vi "CF_TC to PGSQL.vi"(8 "error in (no error)":errorcluster, 9 "calibration string":string, 10 "description string":string, 11 "dbl":dbl[](array[numeric])) -> (0 "error out":errorcluster)   [LabVIEW 2013]
uses:
  postgreSQL-lv/Data.PG/Data.PGSQL.lvclass
panel:
  # "CF TC to PGSQL"
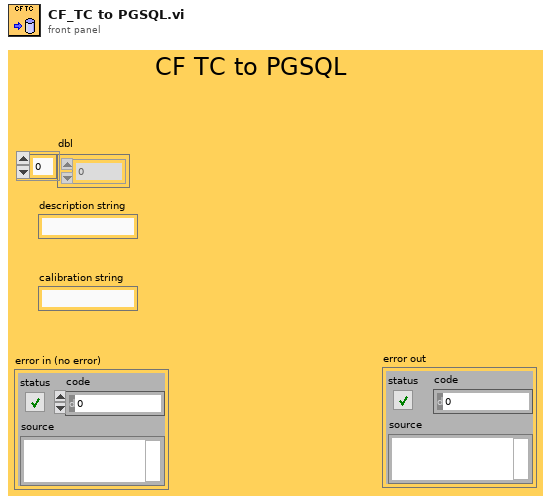
[diagram p1: front panel]
types:
  T1 = cluster{"dbl":dbl[], "description string":string, "calibration string":string}
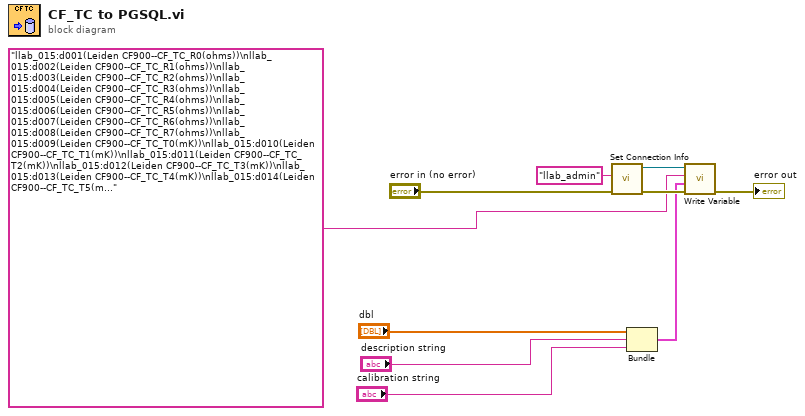
[diagram p0: block diagram]
diagram:
  n1 = call "Set Connection Info.vi"("username"="llab_admin", "error in (no error)"="error in (no error)") -> ("Data.PG out"=w10:refnum<class "Data.PGSQL.lvclass">, "error out"=w9:errorcluster)  [unwired: 7 in]
  n2 = Bundle("dbl"="dbl", "description string"="description string", "calibration string"="calibration string") -> (w7:T1)  [unwired: 1 in]
  n3 = call "Write Variable.vi"("error in (no error)"=w9, "Data"=w7, "variable"="llab_015:d001(Leiden CF900--CF_TC_R0(ohms))\nllab_015:d002(Leiden CF900--CF_TC_R1(ohms))\nllab_015:d003(Leiden CF900--CF_TC_R2(ohms))\nllab_015:d004(Leiden CF900--CF_TC_R3(ohms))\nllab_015:d005(Leiden CF900--CF_TC_R4(ohms))\nllab_015:d006(Leiden CF900--CF_TC_R5(ohms))\nllab_015:d007(Leiden CF900--CF_TC_R6(ohms))\nllab_015:d008(Leiden CF900--CF_TC_R7(ohms))\nllab_015:d009(Leiden CF900--CF_TC_T0(mK))\nllab_015:d010(Leiden CF900--CF_TC_T1(mK))\nllab_015:d011(Leiden CF900--CF_TC_T2(mK))\nllab_015:d012(Leiden CF900--CF_TC_T3(mK))\nllab_015:d013(Leiden CF900--CF_TC_T4(mK))\nllab_015:d014(Leiden CF900--CF_TC_T5(mK))\nllab_015:d015(Leiden CF900--CF_TC_T6(mK))\nllab_015:d016(Leiden CF900--CF_TC_T7(mK))\nllab_015:d017(Leiden CF900--CF_TC_I0(Amp))\nllab_015:d018(Leiden CF900--CF_TC_I1(Amp))\nllab_015:d019(Leiden CF900--CF_TC_I2(Amp))\nllab_015:d020(Leiden CF900--CF_TC_I3(Amp))\nllab_015:v000(Leiden CF900--CF_TC_description())\nllab_015:v001(Leiden CF900--CF_TC_calibration())", "Data.PG in"=w10) -> ("error out"=→"error out":errorcluster)  [unwired: 5 in, 2 out]
